vi "1D Auto Correlation (CDB).vi"(10 "normalization":enum32{"none", "unbiased", "biased"}(ring), 11 "X":cdb[](array[numeric])) -> (0 "error":i32, 3 "Rxx":cdb[](array[numeric]))   [LabVIEW 2024, in "NI_AALPro.lvlib"]
doc: "<p>Computes the autocorrelation of the input sequence <strong>X</strong>. Wire data to the <strong>X</strong> input to determine the polymorphic instance to use or <a href=\"nihelplauncher://docs/csh?context=lvcore_lvhowto_selectingdefaultinstpolyvi\">manually select</a> the instance.</p>"
uses:
  NI_AALPro.lvlib
  <resource>/lvanlys.dll
panel:
  # "1D AutoCorrelation (CDB)"
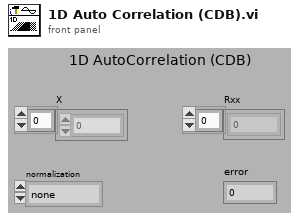
[diagram p1: front panel]
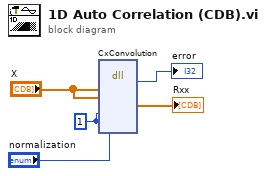
[diagram p0: block diagram]
diagram:
  w1 = 1 ("ConvOrCorr")
  n1 = dll-call lib="C:/Program Files (x86)/National Instruments/LabVIEW 2024/resource/lvanlys.*" fn="CxConvolution"("X"="X", "X"="X", "domain"=w1, "ConvOrCorr"=w1, "norm"="normalization") -> (→"error":i32, "Rxx"=→"Rxx":cdb[])  [unwired: 9 in, 2 out]
